vi "Camera and Joystick Tester.vi"() -> ()   [LabVIEW 2023]
uses:
  Shared Components/Gantry Class/Type Definitions/Virtual Modes.ctl
  Shared Components/Gantry Class/Type Definitions/Init_Modes.ctl
  Shared Components/Gantry Class/Gantry.lvclass
panel:
  in  "Activate Joystick":bool
  in  "Camera Name":string
  in  "Virtual Mode":T1
  in  "HOME?":bool=TRUE
  in  "stop":bool
  out "Image":T2(plugin-control)
  out "error out":errorcluster
  in  "Config Folder":path=path "C:/Users/Admin/Gantry Purdue/pixel-gantry-control/Config"
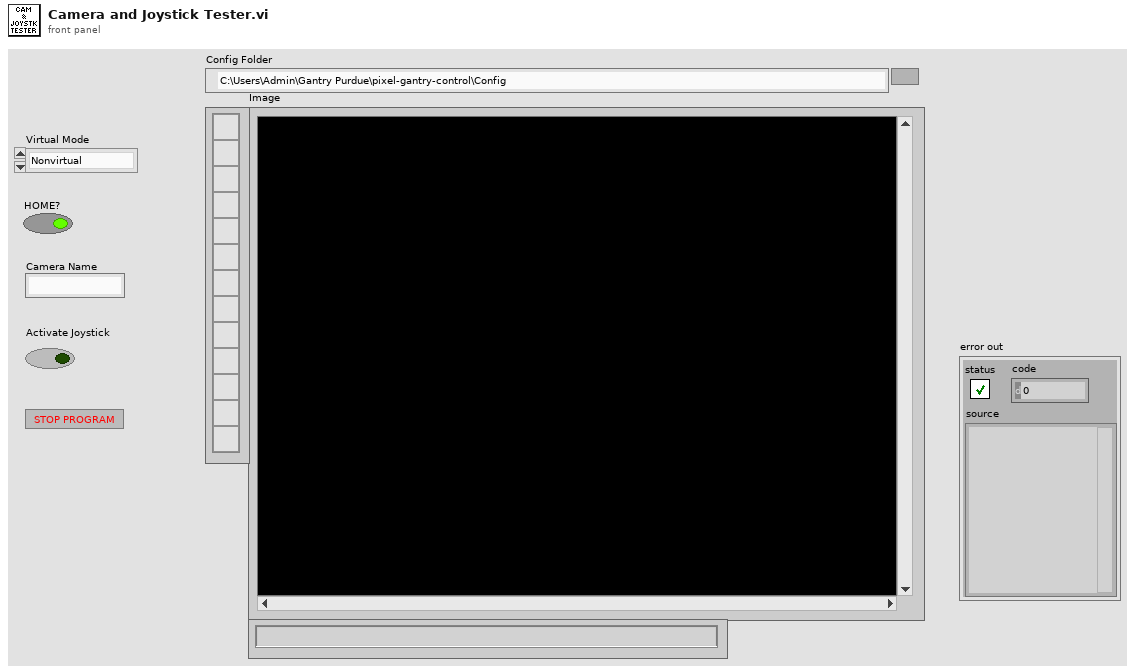
[diagram p1: front panel]
types:
  T1 = typedef "Virtual Modes.ctl" = enum16{"Nonvirtual", "Virtual"}
  T2 = typedef "IMAQ Image.ctl" = refnum<image>
  T3 = typedef "Init_Modes.ctl" = enum16{"Full", "Robot Only", "Dispenser Only", "Cameras Only", "Robot and Cameras", "Robot and Cameras and Dispenser", "Manifold Only"}
  T4 = enum8{"Enabled", "Disabled", "Disabled and Grayed Out"}
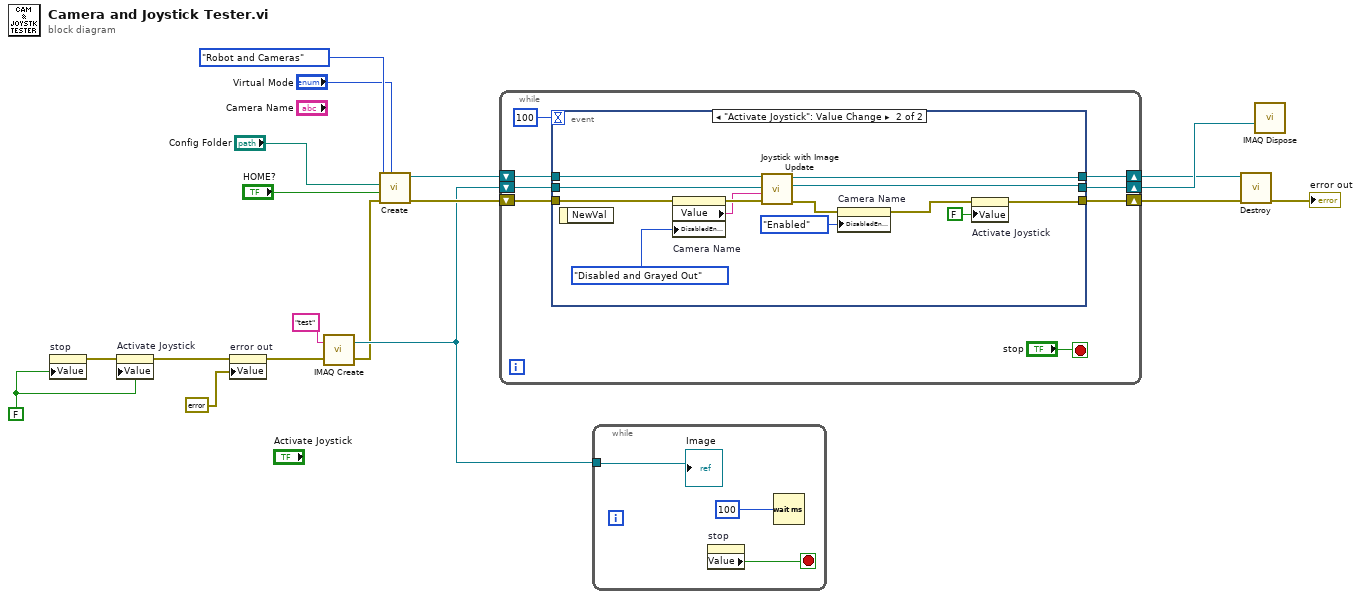
[diagram p0: block diagram]
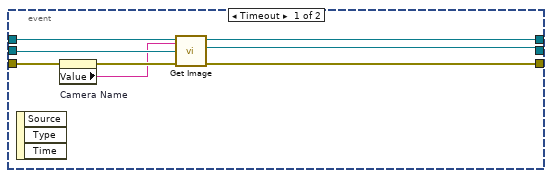
[diagram p2: hidden frame]
diagram:
  w8 = FALSE
  n1 = property on="stop" class="Bool (strict)"("Value"=w8) -> (error out=w9:errorcluster)  [unwired: 2 in, 1 out]
  n2 = property on="Activate Joystick" class="Bool (strict)"(error in=w9, "Value"=w8) -> (error out=w7:errorcluster)  [unwired: 1 in, 1 out]
  n3 = property on="error out" class="Clust (strict)"(error in=w7, "Value"=errorcluster {"status"=FALSE, "code"=0, "source"=""} ("error in (no error)")) -> (error out=w3:errorcluster)  [unwired: 1 in, 1 out]
  n4 = call "IMAQ Create"("Image Name"="test", "error in (no error)"=w3) -> ("New Image"=w5:T2, "error out"=w1:errorcluster)  [unwired: 3 in]
  n5 = call "Create.vi"("Virtual Mode"="Virtual Mode", "error in"=w1, "HOME?"="HOME?", "Project Path"="Config Folder", "Init Mode"=Init_Modes."Robot and Cameras") -> ("error out"=w15:errorcluster, "Gantry out"=w6:refnum<class "Gantry.lvclass">)  [unwired: 5 in]
  n6 = while {
    shift-right: [w24] -> w4
    shift-left: w15 -> [w26]
    shift-right: [w23] -> w10
    shift-left: w6 -> [w22]
    shift-right: [w25] -> w11
    shift-left: w5 -> [w21]
    stop <- "stop" stop-if-true
    n7 = event shown="[1] \"Activate Joystick\": Value Change" {
      selector: _ -> [_ _]
      dyn-events: _ -> [_ _]
      timeout: 100 -> [_ _]
      tunnel: w26 -> [w29 w44]
      tunnel: [w30 w46] -> w25
      tunnel: [w33 w42] -> w24
      tunnel: w22 -> [w34 w47]
      tunnel: [w32 w45] -> w23
      tunnel: w21 -> [w31 w39]
      event Timeout {
        n8 = event-data() -> ()  [unwired: 1 in, 3 out]
        n9 = property on="Camera Name" class="Str"(error in=w29) -> (error out=w28:errorcluster, "Value"=w27:string)  [unwired: 1 in, 1 out]
        n10 = call-dynamic "Get Image.vi"("error in"=w28, "Image In"=w31, "Camera Name"=w27, "Gantry in"=w34) -> ("error out"=w33:errorcluster, "Image Out"=w30:T2, "Gantry out"=w32:refnum<class "Gantry.lvclass">)  [unwired: 4 in, 1 out]
      }
      event "Activate Joystick": Value Change {
        n11 = event-data() -> ()  [unwired: 1 in, 1 out]
        n12 = property on="Camera Name" class="Str"(error in=w44, "DisabledEnum"=T4."Disabled and Grayed Out" ("Disabled")) -> (error out=w43:errorcluster, "Value"=w35:string)  [unwired: 1 in, 1 out]
        n13 = call-dynamic "Joystick with Image Update.vi"("error in (no error)"=w43, "Camera Name"=w35, "Image In"=w39, "Gantry Class in"=w47) -> ("error out"=w38:errorcluster, "Image Out"=w46:T2, "Gantry Class out"=w45:refnum<class "Gantry.lvclass">)  [unwired: 5 in]
        n14 = property on="Camera Name" class="Str"(error in=w38, "DisabledEnum"=T4."Enabled" ("Disabled")) -> (error out=w37:errorcluster)  [unwired: 1 in, 1 out]
        n15 = property on="Activate Joystick" class="Bool (strict)"(error in=w37, "Value"=FALSE ("Activate Joystick")) -> (error out=w42:errorcluster)  [unwired: 1 in, 1 out]
      }
    }
  }
  n16 = while {
    tunnel: w5 -> [w49]
    stop <- w48 stop-if-true
    n17 = property on="stop" class="Bool (strict)"() -> ("Value"=w48:bool)  [unwired: 2 in, 2 out]
    n18 = Wait (ms)(milliseconds to wait=u32 100) -> ()  [unwired: 1 out]
    "Image" <- w49
  }
  n19 = call "Destroy.vi"("error in"=w4, "Gantry Class in"=w10) -> ("error out"=→"error out":errorcluster)  [unwired: 9 in]
  n20 = call "IMAQ Dispose"("Image"=w11) -> ()  [unwired: 5 in, 1 out]
